vi "Main5.vi"(4 "מק\"ט המכלל":string, 5 "מספר סידורי":string, 7 "מפעיל":string="ANS", 8 "error":errorcluster, 11 "Path for Log":path) -> (0 "error IO":errorcluster)   [LabVIEW 2015]
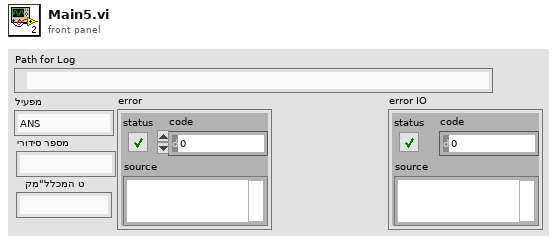
[diagram p1: front panel]
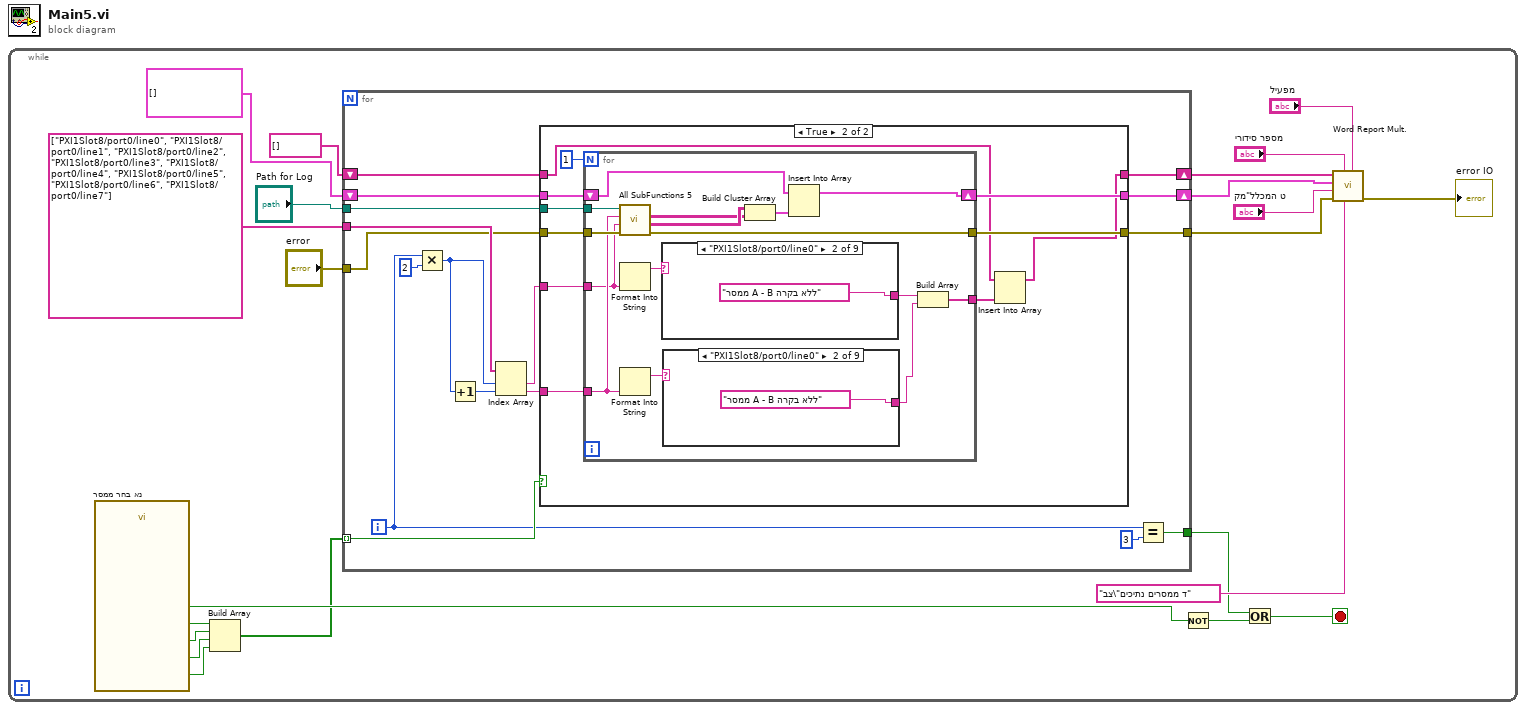
[diagram p0: block diagram]
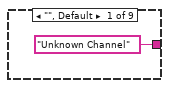
[diagram p3: hidden frame]
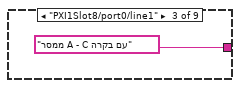
[diagram p4: hidden frame]
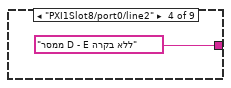
[diagram p5: hidden frame]
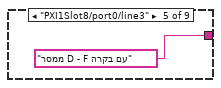
[diagram p6: hidden frame]
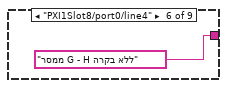
[diagram p7: hidden frame]
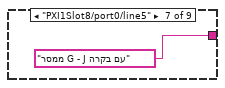
[diagram p8: hidden frame]
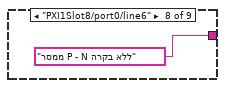
[diagram p9: hidden frame]
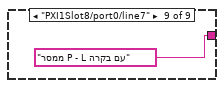
[diagram p10: hidden frame]
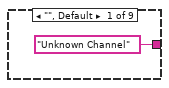
[diagram p11: hidden frame]
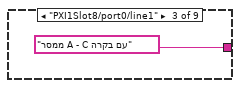
[diagram p12: hidden frame]
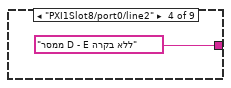
[diagram p13: hidden frame]
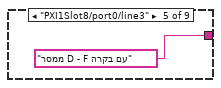
[diagram p14: hidden frame]
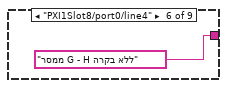
[diagram p15: hidden frame]
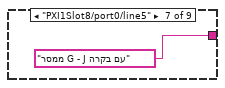
[diagram p16: hidden frame]
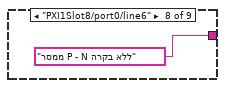
[diagram p17: hidden frame]
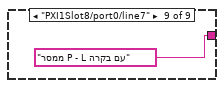
[diagram p18: hidden frame]
diagram:
  n1 = while {
    stop <- w2 stop-if-true
    n2 = call "נא בחר ממסר.vi"() -> ("P - N/L"=w19:bool, "G - H/J"=w18:bool, "D - E/F"=w17:bool, "A - B/C"=w16:bool, "OK"=w22:bool)  [unwired: 13 in, 2 out]
    n3 = Build Array(w16, w17, w18, w19) -> (w21:bool[])
    n4 = for {
      tunnel: w21 -> [w39] mode=indexing
      tunnel: tag[] ["PXI1Slot8/port0/line0", "PXI1Slot8/port0/line1", "PXI1Slot8/port0/line2", "PXI1Slot8/port0/line3", "PXI1Slot8/port0/line4", "PXI1Slot8/port0/line5", "PXI1Slot8/port0/line6", "PXI1Slot8/port0/line7"] -> [w38]
      tunnel: "Path for Log" -> [w32]
      tunnel: [w31] -> w6
      tunnel: "error" -> [w30]
      shift-right: [w28] -> w8
      shift-left: cluster{"appended array":string[][]}[] [] ("array of clusters") -> [w29]
      shift-right: [w26] -> w4
      shift-left: string[] [] ("Array 2") -> [w27]
      tunnel: [w23] -> w1
      i -> [w25]
      n5 = Multiply(x=w25, y=2) -> (x*y=w36:i32)
      n6 = Increment(x=w36) -> (x+1=w35:i32)
      n7 = Index Array(array=w38, index #1=w36, index #2=w35) -> (element #1=w34:tag, element #2=w33:tag)
      n8 = case shown="True" w39 {
        tunnel: w34 -> [_ w46]
        tunnel: w33 -> [_ w45]
        tunnel: w32 -> [_ w53]
        tunnel: [w42 w52] -> w31
        tunnel: w30 -> [w42 w51]
        tunnel: w29 -> [w41 w50]
        tunnel: [w41 w49] -> w28
        tunnel: w27 -> [w40 w48]
        tunnel: [w40 w47] -> w26
        frame False {
        }
        frame True {
          n9 = for {
            N: 1 -> [_]
            tunnel: w53 -> [w68]
            tunnel: [w67] -> w52
            tunnel: w51 -> [w66]
            shift-right: [w62] -> w49
            shift-left: w50 -> [w64]
            tunnel: w46 -> [w59]
            tunnel: w45 -> [w60]
            tunnel: [w61] -> w44
            n10 = call "All SubFunctions 5.vi"("error"=w66, "lines 1"=w59, "lines"=w60, "Path for Log"=w68) -> ("error IO"=w67:errorcluster, "appended array 1"=w57:string[][], "appended array"=w56:string[][])  [unwired: 5 in]
            n11 = Format Into String(w59) -> (resulting string=w65:string)  [unwired: 3 in, 1 out]
            n12 = Format Into String(w60) -> (resulting string=w54:string)  [unwired: 3 in, 1 out]
            n13 = case shown="\"PXI1Slot8/port0/line0\"" w65 {
              tunnel: ["Unknown Channel" "ממסר A - B ללא בקרה" "ממסר A - C עם בקרה" "ממסר D - E ללא בקרה" "ממסר D - F עם בקרה" "ממסר G - H ללא בקרה" "ממסר G - J עם בקרה" "ממסר P - N ללא בקרה" "ממסר P - L עם בקרה"] -> w58
              frame "", Default {
              }
              frame "PXI1Slot8/port0/line0" {
              }
              frame "PXI1Slot8/port0/line1" {
              }
              frame "PXI1Slot8/port0/line2" {
              }
              frame "PXI1Slot8/port0/line3" {
              }
              frame "PXI1Slot8/port0/line4" {
              }
              frame "PXI1Slot8/port0/line5" {
              }
              frame "PXI1Slot8/port0/line6" {
              }
              frame "PXI1Slot8/port0/line7" {
              }
            }
            n14 = case shown="\"PXI1Slot8/port0/line0\"" w54 {
              tunnel: ["Unknown Channel" "ממסר A - B ללא בקרה" "ממסר A - C עם בקרה" "ממסר D - E ללא בקרה" "ממסר D - F עם בקרה" "ממסר G - H ללא בקרה" "ממסר G - J עם בקרה" "ממסר P - N ללא בקרה" "ממסר P - L עם בקרה"] -> w55
              frame "", Default {
              }
              frame "PXI1Slot8/port0/line0" {
              }
              frame "PXI1Slot8/port0/line1" {
              }
              frame "PXI1Slot8/port0/line2" {
              }
              frame "PXI1Slot8/port0/line3" {
              }
              frame "PXI1Slot8/port0/line4" {
              }
              frame "PXI1Slot8/port0/line5" {
              }
              frame "PXI1Slot8/port0/line6" {
              }
              frame "PXI1Slot8/port0/line7" {
              }
            }
            n15 = Build Cluster Array(w57, w56) -> (w63:cluster{"appended array":string[][]}[])
            n16 = Insert Into Array(array=w64, new element=w63) -> (w62:cluster{"appended array":string[][]}[])  [unwired: 1 in]
            n17 = Build Array(w58, w55) -> (w61:string[])
          }
          n18 = Insert Into Array(array=w48, new element=w44) -> (w47:string[])  [unwired: 1 in]
        }
      }
      n19 = Equal?(x=w25, y=3) -> (x = y?=w23:bool)
    }
    n20 = Not(x=w22) -> (.not. x?=w3:bool)
    n21 = Or(x=w1, y=w3) -> (x .or. y?=w2:bool)
    n22 = call "Word Report Mult..vi"("מפעיל"="מפעיל", "שם הצב\"ד"="צב\"ד ממסרים נתיכים", "מספר סידורי"="מספר סידורי", "error in (no error)"=w6, "מק\"ט המכלל"="מק\"ט המכלל", "Array of Items"=w8, "Elements"=w4) -> ("error out"=→"error IO":errorcluster)  [unwired: 4 in]
  }
